vi "generateMEM.vi"() -> ()   [LabVIEW 2017]
uses:
  <vilib>/Utility/file.llb/Read Delimited Spreadsheet (I64).vi
  <vilib>/Utility/file.llb/Write Delimited Spreadsheet (string).vi
panel:
  out "appended path":path
  in  "saved ch list":u16[](array[numeric])=[0, 2, 4, 6]
  in  "file path (dialog if empty)":path=path "G:/tdc/2017/code_density_rom.mem"
  out "size(s)":i32[](array[numeric])=[2048, 128]
  out "cal":u32[][](graph)
  in  "通道数量":i32=128
  in  "ch list":u16[](array[numeric])=[0, 1, 2, 3, 4, 5, 6, 7]
  in  "codeDensity":path=path "G:/tdc/2017/test_20240327_123704_codeDensity.csv"
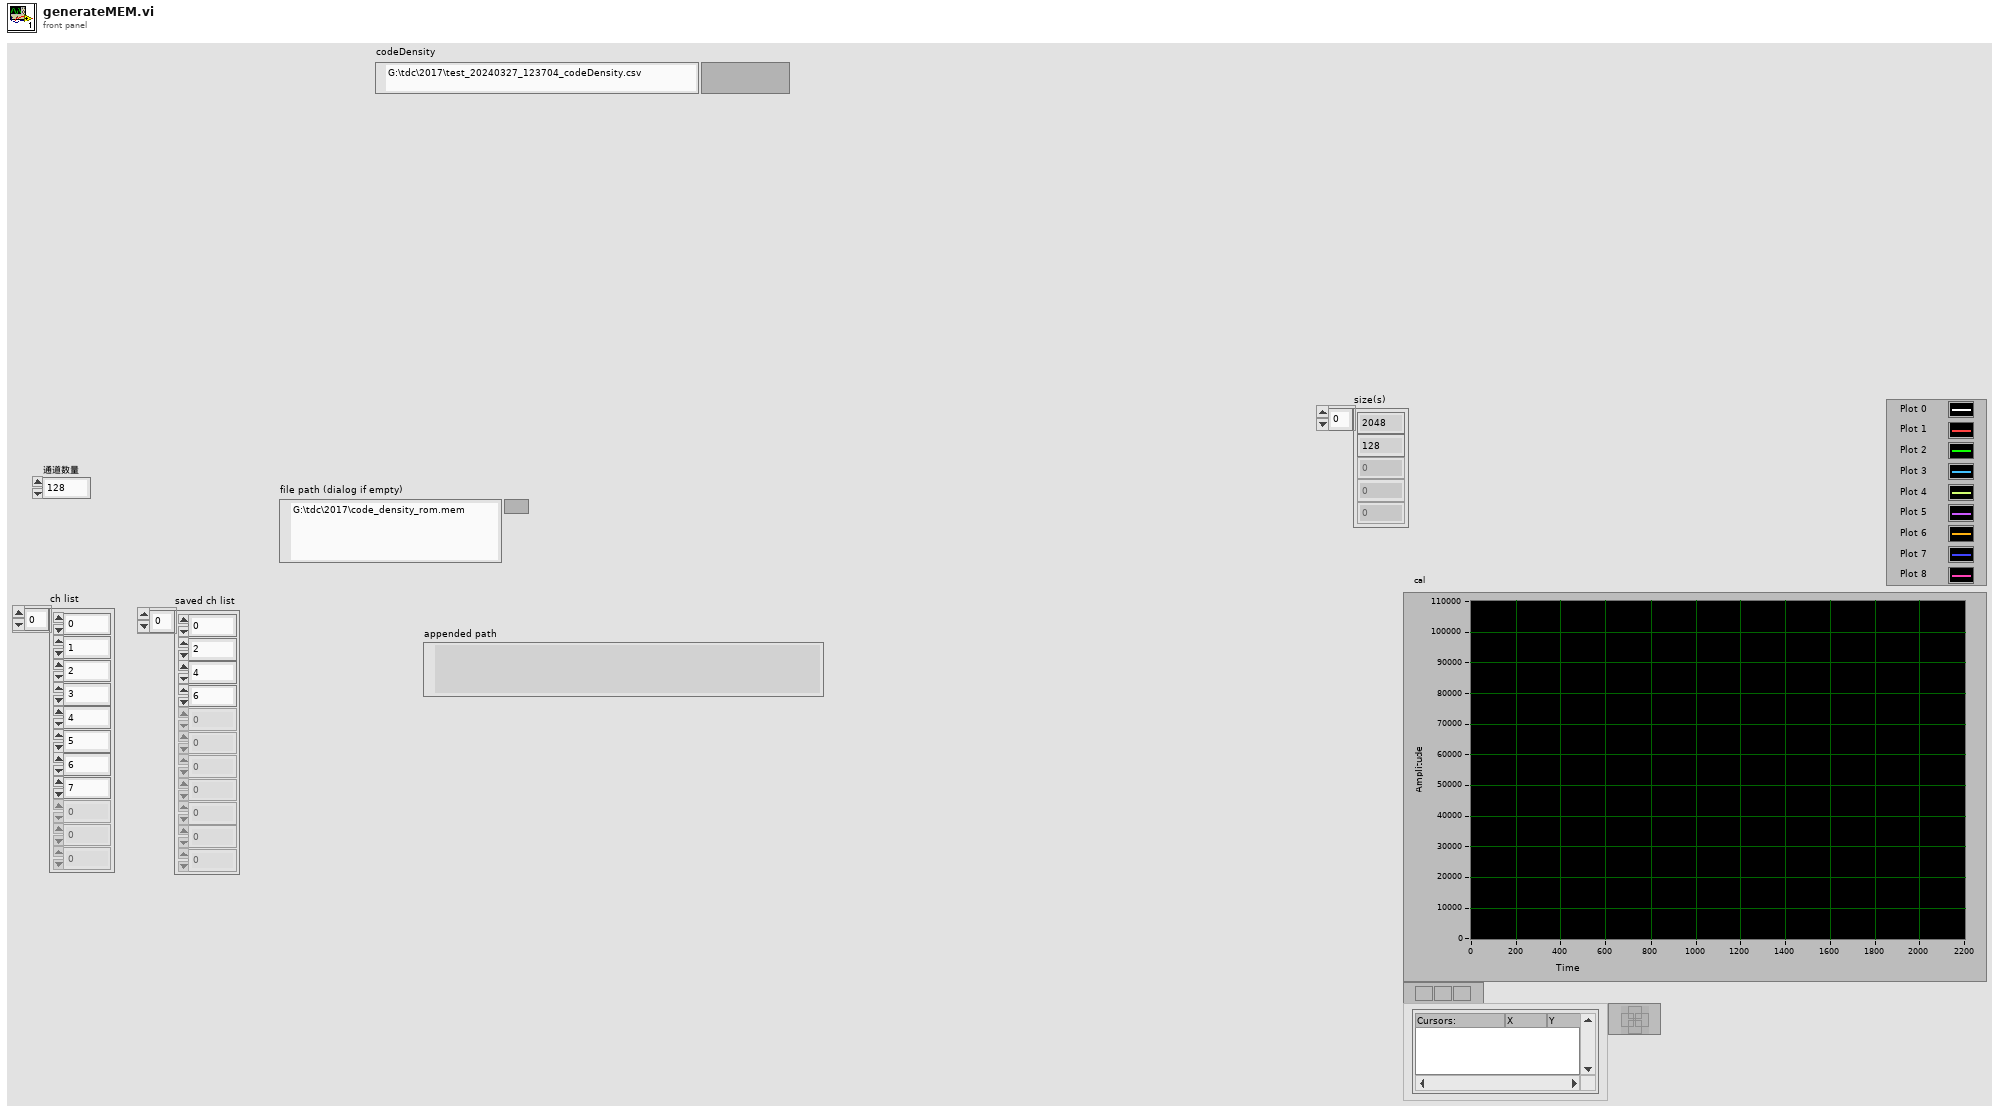
[diagram p1: front panel]
types:
  T1 = enum16{"open", "replace", "create", "open or create", "replace or create", "replace or create with confirmation"}
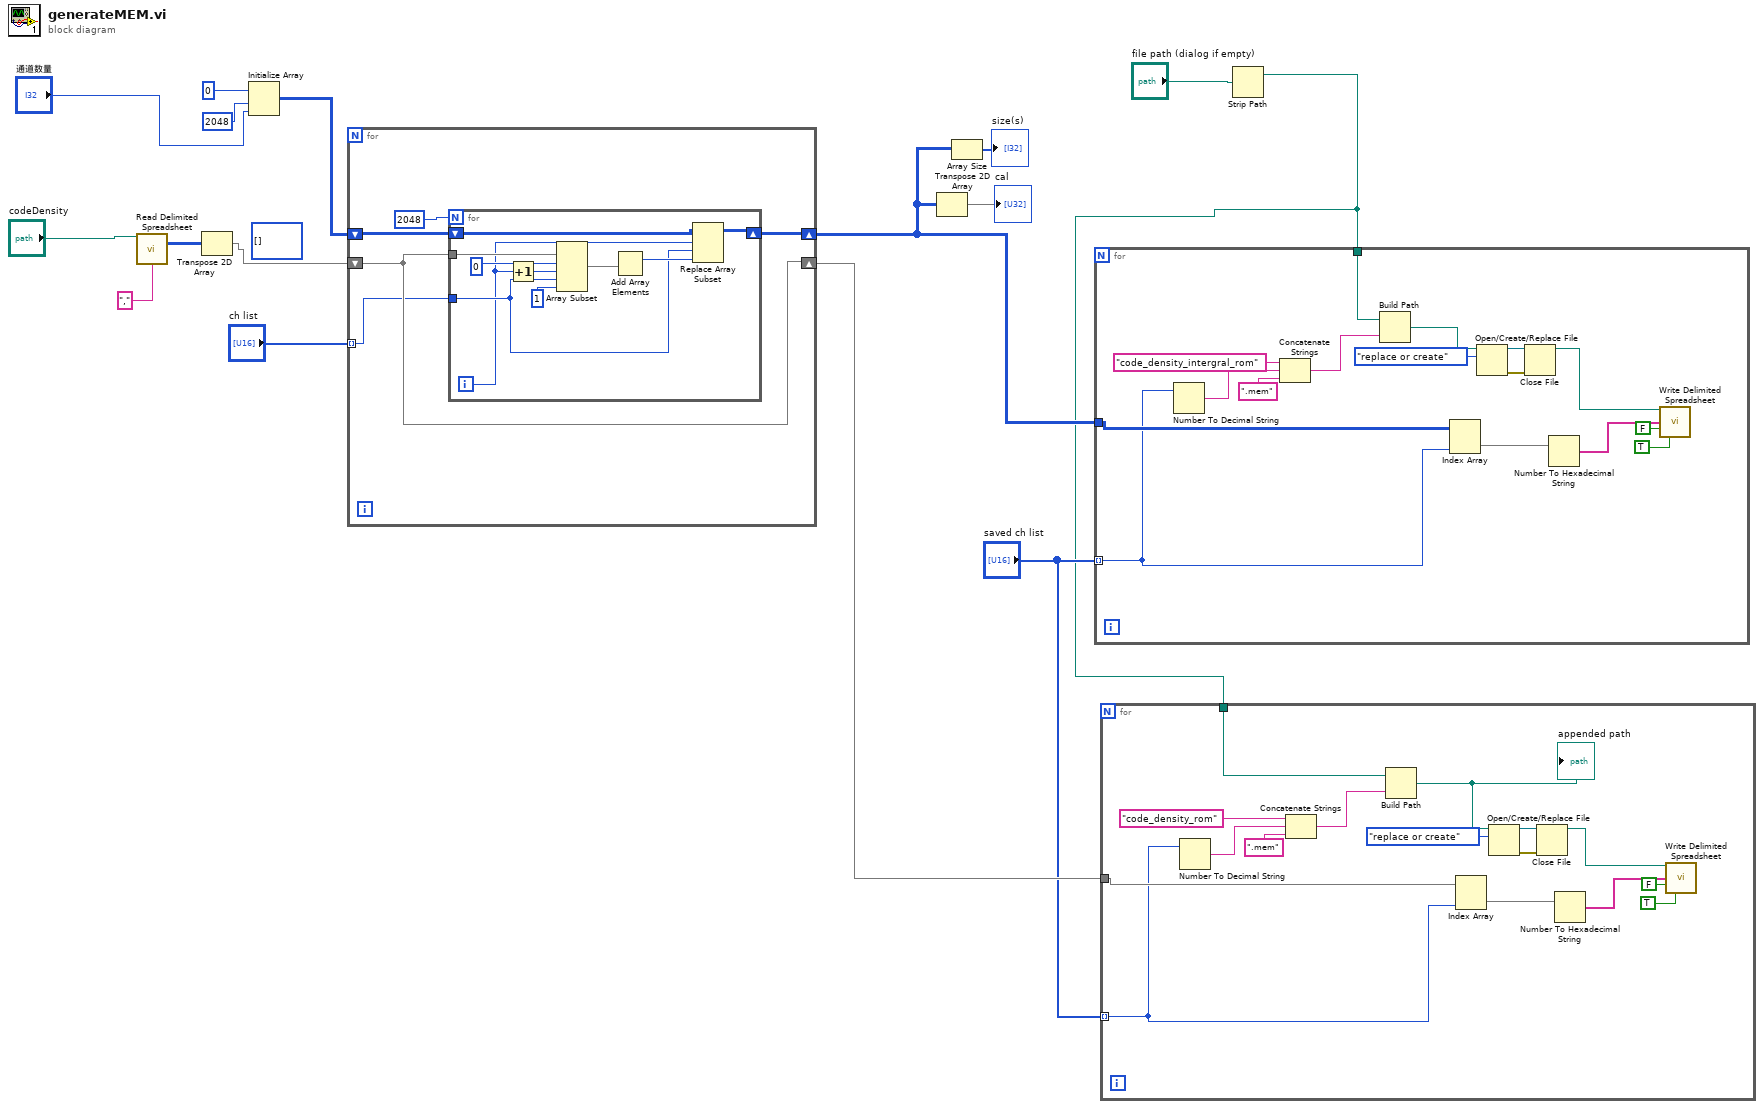
[diagram p0: block diagram]
diagram:
  (unwired) i64[][] []
  n1 = call-poly <vilib>:"Read Delimited Spreadsheet.vi"("file path (dialog if empty)"="codeDensity", "delimiter (\\t)"="," ("delimiter (\\t)")) -> ("all rows"=w16:i64[][])  [unwired: 8 in, 5 out]
  n2 = Transpose 2D Array(2D array=w16) -> (transposed array=w8:i64[][])
  n3 = Initialize Array(u32 0 ("element"), 2048 ("dimension size"), "通道数量") -> (w9:u32[][])
  n4 = for {
    shift-right: [w19] -> w5
    shift-left: w9 -> [w20]
    shift-right: [w18] -> w4
    shift-left: w8 -> [w18]
    tunnel: "ch list" -> [w17] mode=indexing
    n5 = for {
      N: 2048 -> [_]
      tunnel: w18 -> [w31]
      tunnel: w17 -> [w24]
      shift-right: [w26] -> w19
      shift-left: w20 -> [w27]
      i -> [w23]
      n6 = Increment(x=w23) -> (x+1=w22:i32)
      n7 = Array Subset(array=w31, index (row)=0 ("索引"), length (row)=w22, index (col)=w24, length (col)=1 ("长度")) -> (w28:i64[][])
      n8 = Add Array Elements(numeric array=w28) -> (sum=w25:i64)
      n9 = Replace Array Subset(array=w27, new element=w25, index (row)=w23, index (col)=w24) -> (w26:u32[][])
    }
  }
  n10 = Transpose 2D Array(2D array=w5) -> (transposed array=→"cal":u32[][])
  n11 = Array Size(array=w5) -> (size(s)=→"size(s)":i32[])
  n12 = Strip Path(path="file path (dialog if empty)") -> (stripped path=w1:path)  [unwired: 1 out]
  n13 = for {
    tunnel: w5 -> [w41]
    tunnel: "saved ch list" -> [w38] mode=indexing
    tunnel: w1 -> [w32]
    n14 = Number To Decimal String(number=w38) -> (decimal integer string=w46:string)  [unwired: 1 in]
    n15 = Concatenate Strings("code_density_intergral_rom", w46, ".mem") -> (w44:string)
    n16 = Build Path(base path=w32, name or relative path=w44) -> (appended path=w34:path)
    n17 = Index Array(array=w41, index (col)=w38) -> (element=w40:u32[])  [unwired: 1 in]
    n18 = Open/Create/Replace File(file path (use dialog)=w34, operation (0:open)=T1."replace or create") -> (refnum out=w35:refnum<file>, error out=w36:errorcluster)  [unwired: 4 in, 1 out]
    n19 = Close File(refnum=w35, error in=w36) -> (path=w33:path)  [unwired: 1 out]
    n20 = Number To Hexadecimal String(2:w40) -> (0:w39:string[])  [unwired: 1 in]
    n21 = call-poly <vilib>:"Write Delimited Spreadsheet.vi"("file path (dialog if empty)"=w33, "1D data"=w39, "append to file? (new file:F)"=FALSE, "transpose? (no:F)"=TRUE) -> ()  [unwired: 10 in, 2 out]
  }
  n22 = for {
    tunnel: w4 -> [w56]
    tunnel: w1 -> [w63]
    tunnel: "saved ch list" -> [w53] mode=indexing
    n23 = Number To Decimal String(number=w53) -> (decimal integer string=w61:string)  [unwired: 1 in]
    n24 = Concatenate Strings("code_density_rom", w61, ".mem") -> (w59:string)
    n25 = Build Path(base path=w63, name or relative path=w59) -> (appended path=w49:path)
    "appended path" <- w49
    n26 = Index Array(array=w56, index (col)=w53) -> (element=w55:i64[])  [unwired: 1 in]
    n27 = Open/Create/Replace File(file path (use dialog)=w49, operation (0:open)=T1."replace or create") -> (refnum out=w52:refnum<file>, error out=w51:errorcluster)  [unwired: 4 in, 1 out]
    n28 = Close File(refnum=w52, error in=w51) -> (path=w48:path)  [unwired: 1 out]
    n29 = Number To Hexadecimal String(2:w55) -> (0:w54:string[])  [unwired: 1 in]
    n30 = call-poly <vilib>:"Write Delimited Spreadsheet.vi"("file path (dialog if empty)"=w48, "1D data"=w54, "append to file? (new file:F)"=FALSE, "transpose? (no:F)"=TRUE) -> ()  [unwired: 10 in, 2 out]
  }
